vi "Gasteiler_Nullpunkt.vi"   [LabVIEW 2020, in "Linearisierung v2.lvlib"]
uses:
  Linearisierung v2.lvlib
  Gasteiler/Aktionen FGV Gasteiler Daten.ctl
  Gasteiler/AK-Komm Gasteiler/Aktionen AK Komm.ctl
  Gasteiler/AK-Komm Gasteiler/Alter Gasteiler/Aktionen AK Komm_ALT.ctl
  Gasteiler/Horiba/Aktion Befehl.ctl
  Gasteiler/AK-Komm Gasteiler/AK Komm Gasteiler.lvlib
  Gasteiler/Horiba/Horiba GDC.lvlib
  Gasteiler/AK-Komm Gasteiler/Alter Gasteiler/Alter Gasteiler.lvlib
  Gasteiler/Gasteiler.lvlib
  Gasteiler/HovaCAL_Interface/Kommunikation/Kommunikation.lvlib
types:
  T1 = typedef "Linearisierung v2.lvlib/Gasteiler.lvlib/Aktionen FGV Gasteiler Daten.ctl" = enum16{"lesen", "Gasteiler Daten", "Seriellen Param.", "MB-Endwert", "laden", "speichern", "Anforderung", "TCP", "Aufzeichnung Start"}
  T2 = typedef "Linearisierung v2.lvlib/GasteilerType.ctl" = u16
  T3 = typedef "Linearisierung v2.lvlib/Gasteiler.lvlib/AK Komm Gasteiler.lvlib/Aktionen AK Komm.ctl" = enum16{"lesen", "initialisieren", "beenden", "Status", "SMAN", "SREM", "STBY", "ASTF", "ASTZ", "SLST", "AGAT", "EGAK", "AGAK", "AKAK", "ADRU", "SKOP", "SVSA", "SVSZ", "SONO", "SAIR", "SNOX", "ANOX", "SSPL", "SRUC", "SLIN", "ALST", "ETYP", "SVIO", "LCYL", "CCYL", "DCYL", "SCYL", "GCYL", "DRGV", "DRDC"}
  T4 = typedef "Linearisierung v2.lvlib/Gasteiler.lvlib/AK Komm Gasteiler.lvlib/Alter Gasteiler.lvlib/Aktionen AK Komm_ALT.ctl" = enum16{"lesen", "initialisieren", "beenden", "SRES", "STBY", "SREM", "SMAN", "SLIN", "SLCH", "SLST", "SSPL", "AGAT", "ALST", "ASTZ", "ASTF", "AGAK", "EGAK"}
  T5 = typedef "Linearisierung v2.lvlib/Gasteiler.lvlib/Horiba GDC.lvlib/Aktion Befehl.ctl" = enum16{"lesen", "initialisieren", "Beenden", "Standby", "GD/CC", "Info", "Flow", "Alarm", "GD parameter", "GD point", "Durchfluss", "Spuelen1", "Spuelen1 On", "Spuelen1Off", "Spuelen2", "Ventil-Abfrage", "Reset"}
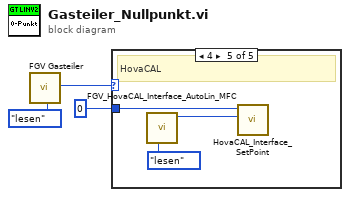
[diagram p0: block diagram]
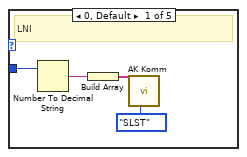
[diagram p2: hidden frame]
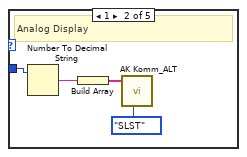
[diagram p3: hidden frame]
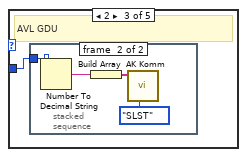
[diagram p4: hidden frame]
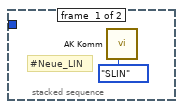
[diagram p5: hidden frame]
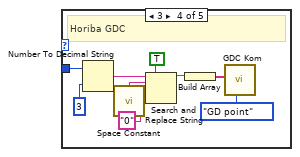
[diagram p6: hidden frame]
diagram:
  n1 = call "FGV Gasteiler.vi"("Aktionen"=Aktionen_FGV_Gasteiler_Daten."lesen") -> ("Gasteiler Type"=w1:T2)  [unwired: 11 in, 7 out]
  n2 = case shown="4" w1 {
    tunnel: 0 ("Punkt") -> [w4 w10 w12 w24 w27]
    frame 0, Default {
      # "LNI"
      n3 = Number To Decimal String(number=w4) -> (decimal integer string=w7:string)  [unwired: 1 in]
      n4 = Build Array(w7) -> (w6:string[])
      n5 = call "AK Komm.vi"("Aktionen"=Aktionen_AK_Komm."SLST", "Daten"=w6) -> ()  [unwired: 3 in, 7 out]
    }
    frame 1 {
      # "Analog Display"
      n6 = Number To Decimal String(number=w10) -> (decimal integer string=w11:string)  [unwired: 1 in]
      n7 = Build Array(w11) -> (w9:string[])
      n8 = call "AK Komm_ALT.vi"("Aktionen_ALT"=Aktionen_AK_Komm_ALT."SLST", "Daten"=w9) -> ()  [unwired: 5 in, 5 out]
    }
    frame 2 {
      # "AVL GDU"
      n9 = stacked-sequence {
        tunnel: w12 -> [_ w16]
        frame #0 {
          # "#Neue_LIN"
          n10 = call "AK Komm.vi"("Aktionen"=Aktionen_AK_Komm."SLIN") -> ()  [unwired: 4 in, 7 out]
        }
        frame #1 {
          n11 = Number To Decimal String(number=w16) -> (decimal integer string=w17:string)  [unwired: 1 in]
          n12 = Build Array(w17) -> (w15:string[])
          n13 = call "AK Komm.vi"("Aktionen"=Aktionen_AK_Komm."SLST", "Daten"=w15) -> ()  [unwired: 3 in, 7 out]
        }
      }
    }
    frame 3 {
      # "Horiba GDC"
      n14 = Number To Decimal String(number=w24, width (-)=i16 3 ("Breite (-)")) -> (decimal integer string=w19:string)
      n15 = call <vilib>:"Space Constant.vi"() -> ("String"=w23:string)
      n16 = Search and Replace String(replace all?=TRUE ("Alle ersetzen? (F)"), input string=w19, search string=w23, replace string="0" ("Ersetzungs-String (\"\")")) -> (result string=w20:string)  [unwired: 4 in, 3 out]
      n17 = Build Array(w20) -> (w25:string[])
      n18 = call "GDC Kom.vi"("Befehl"=Aktion_Befehl."GD point", "Daten"=w25) -> ()  [unwired: 3 in, 7 out]
    }
    frame 4 {
      # "HovaCAL"
      n19 = call "FGV_HovaCAL_Interface_AutoLin_MFC.vi"("Aktion"=enum16{"lesen", "schreiben"}."lesen") -> ("AutoLin MFC out"=w28:u16)  [unwired: 7 in, 3 out]
      n20 = call "HovaCAL_Interface_SetPoint.vi"("AutoLin MFC Index"=w28, "Konzentration"=w27) -> ()  [unwired: 9 in, 1 out]
    }
  }
